vi "Get Child Nodes.vi"(8 "error in":errorcluster, 11 "Node":refnum<k20>) -> (0 "error out":errorcluster, 3 "Child Nodes":refnum<k20>[](array[refnum]))   [LabVIEW 2024, in "Config File Parser.lvlib"]
uses:
  Config File Parser.lvlib
  <vilib>/xml/NI_XML.lvlib
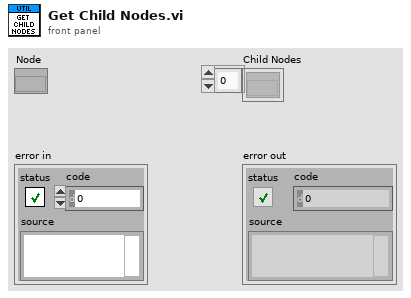
[diagram p1: front panel]
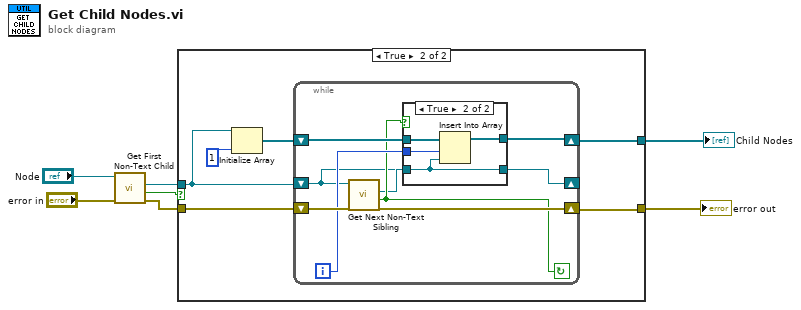
[diagram p0: block diagram]
diagram:
  n1 = call <vilib>:"Get First Non-Text Child.vi"("error in (no error)"="error in", "node in"="Node") -> ("error out"=w5:errorcluster, "found child node?"=w1:bool, "child node"=w2:refnum<k20>)  [unwired: 6 in, 1 out]
  n2 = case shown="True" w1 {
    tunnel: w2 -> [_ w10]
    tunnel: [_ w9] -> w4
    tunnel: w5 -> [w8 w14]
    tunnel: [w8 w13] -> w6
    frame False {
    }
    frame True {
      n3 = Initialize Array(w10, 1 ("dimension size")) -> (w11:refnum<k20>[])
      n4 = while {
        shift-right: [w16] -> _
        shift-left: w10 -> [w15]
        shift-right: [w20] -> w9
        shift-left: w11 -> [w21]
        shift-right: [w22] -> w13
        shift-left: w14 -> [w23]
        i -> [w19]
        stop <- w18 continue-if-true
        n5 = call <vilib>:"Get Next Non-Text Sibling.vi"("error in (no error)"=w23, "node in"=w15) -> ("error out"=w22:errorcluster, "found sibling node?"=w18:bool, "sibling node"=w17:refnum<k20>)  [unwired: 6 in, 1 out]
        n6 = case shown="True" w18 {
          tunnel: w21 -> [w25 w29]
          tunnel: [w25 w28] -> w20
          tunnel: w19 -> [_ w27]
          tunnel: w17 -> [_ w26]
          tunnel: [w24 w26] -> w16
          tunnel: w15 -> [w24 _]
          frame False {
          }
          frame True {
            n7 = Insert Into Array(array=w29, index=w27, new element=w26) -> (w28:refnum<k20>[])
          }
        }
      }
    }
  }
  "Child Nodes" <- w4
  "error out" <- w6
